vi "Result.vi"(8 "error in (no error)":errorcluster, 10 "Results":T1={"Name"="", "Description"="", "Status"=enum."Passed", "Result Type"=enum."Test Suite", "Execution Time"=0.0, "Data"={"Expected"=variant, "Actual"=variant, "Delta"=variant}}, 11 "Result Model In":refnum<class "Result Model.lvclass">) -> (0 "error out":errorcluster, 3 "Result Model Out":refnum<class "Result Model.lvclass">)   [LabVIEW 2020, in "Result Model.lvclass"]
uses:
  Result Model.lvclass
  Core/Result/Result.ctl
  Core/Result/Status.ctl
  Core/Result/Type.ctl
  Result Model.lvclass/Result Model.ctl
  <vilib>/Utility/miscctls.llb/LVMapReplaceAction.ctl
  Core/Result/Result.lvlib
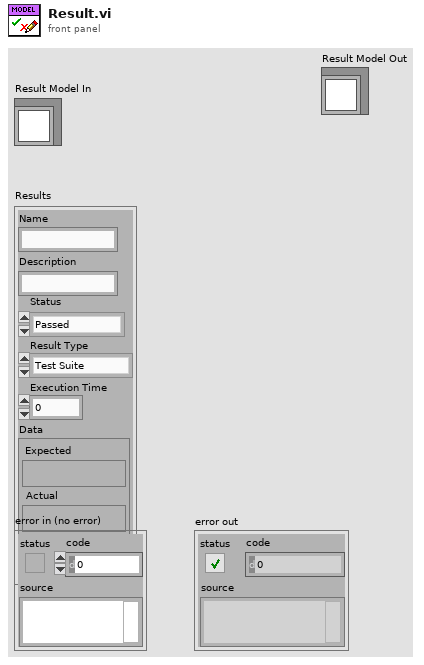
[diagram p1: front panel]
types:
  T1 = typedef "Result.lvlib/Result.ctl" = cluster{"Name":string, "Description":string, "Status":T2, "Result Type":T3, "Execution Time":dbl, "Data":cluster{"Expected":variant, "Actual":variant, "Delta":variant}}
  T2 = typedef "Result.lvlib/Status.ctl" = enum16{"", "Passed", "Failed", "Error", "Skipped", "Setup Error", "Broken", "Teardown Error"}
  T3 = typedef "Result.lvlib/Type.ctl" = enum16{"Test Case", "Test Suite", "Test Run", "Pass", "Fail", "Skip", "Pass if", "Fail if", "Pass if Error", "Fail if Error", "Pass if Equal", "Fail if Equal"}
  T4 = cluster{"Expected":variant, "Actual":variant, "Delta":variant}
  T5 = typedef "LVMapReplaceAction.ctl" = enum32{"Modify Entry only if found", "Add or Modify Entry", "Delete Entry"}
  T6 = cluster{"Result Type":T3, "Status":T2, "Description":string, "Data":cluster{"Expected":variant, "Actual":variant, "Delta":variant}}
  T7 = map{string, cluster{"Result Type":T3, "Status":T2, "Description":string, "Data":cluster{"Expected":variant, "Actual":variant, "Delta":variant}}[]}
  T8 = cluster{"Result Type":T3, "Status":T2, "Description":string, "Data":cluster{"Expected":variant, "Actual":variant, "Delta":variant}}[]
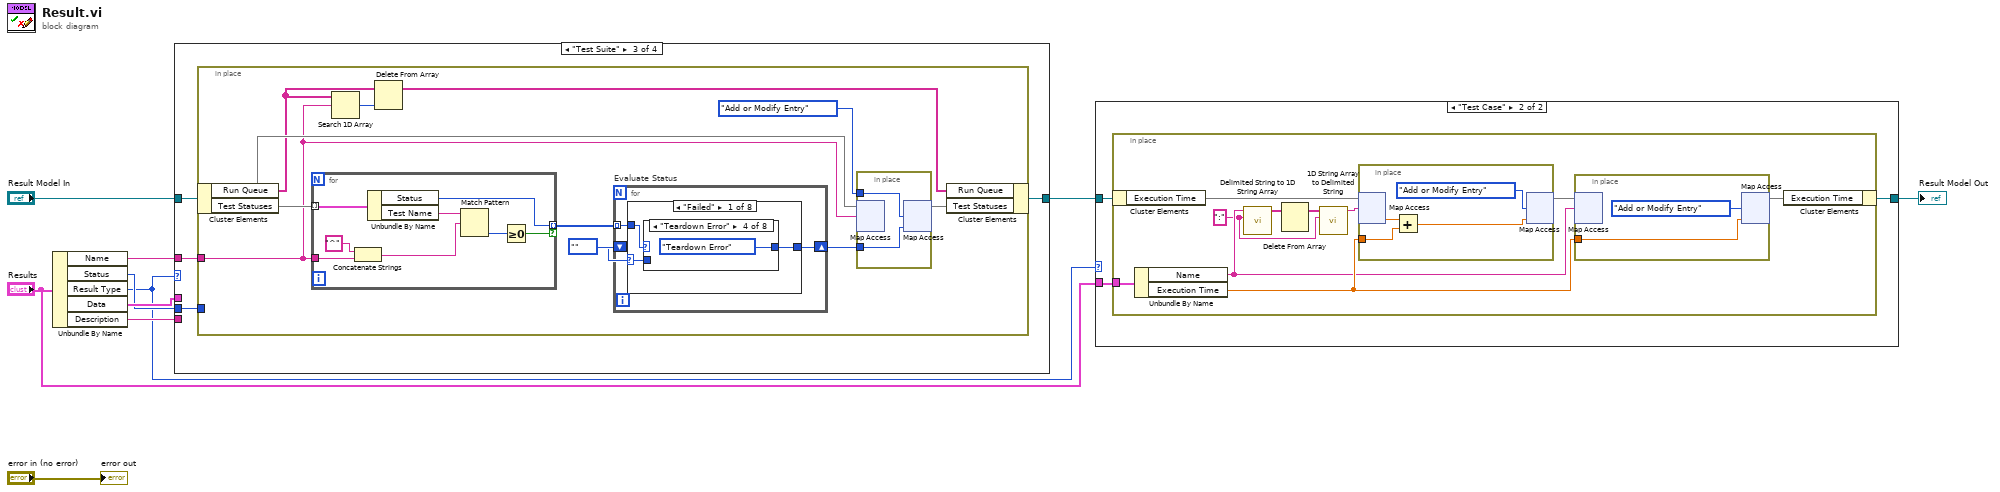
[diagram p0: block diagram]
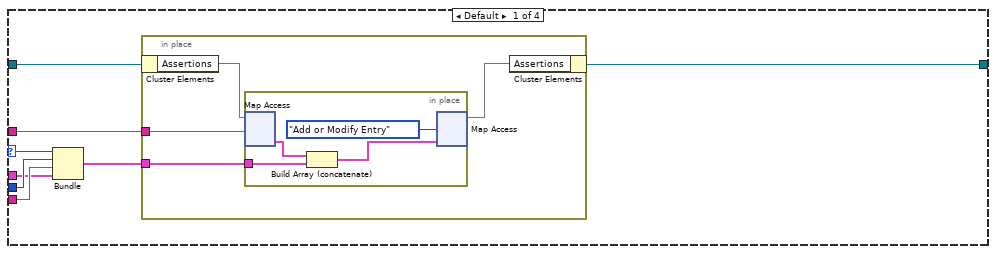
[diagram p2: hidden frame]
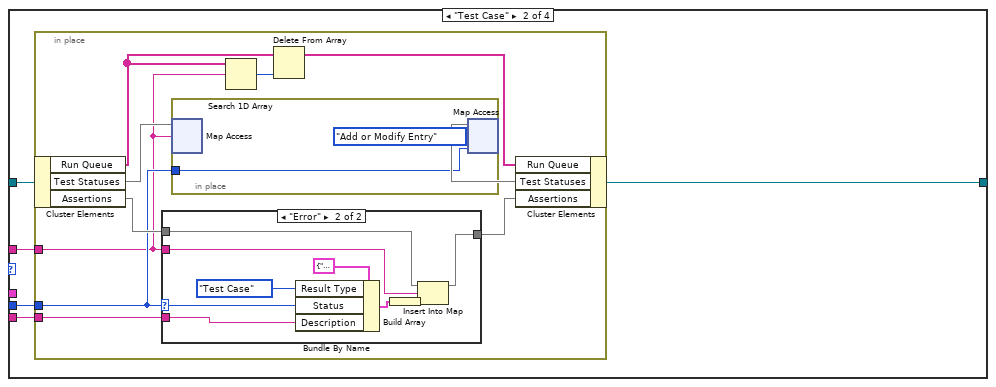
[diagram p3: hidden frame]
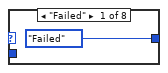
[diagram p5: hidden frame]
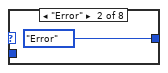
[diagram p6: hidden frame]
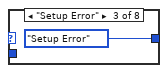
[diagram p7: hidden frame]
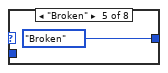
[diagram p8: hidden frame]
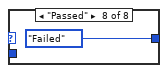
[diagram p11: hidden frame]
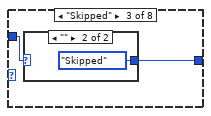
[diagram p13: hidden frame]
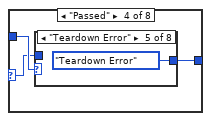
[diagram p15: hidden frame]
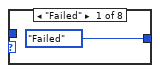
[diagram p16: hidden frame]
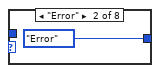
[diagram p17: hidden frame]
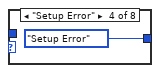
[diagram p19: hidden frame]
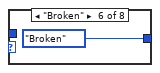
[diagram p20: hidden frame]
diagram:
  n1 = Unbundle By Name("Results") -> ("Name"=w2:string, "Status"=w3:T2, "Result Type"=w1:T3, "Data"=w5:T4, "Description"=w4:string)
  n2 = case shown="\"Test Suite\"" w1 {
    selector: w1 -> [w15 _ _ _]
    tunnel: w2 -> [w16 w31 w57 _]
    tunnel: w3 -> [w14 w30 w56 _]
    tunnel: w4 -> [w17 w27 _ _]
    tunnel: "Result Model In" -> [w13 w29 w55 w126]
    tunnel: [w12 w28 w54 w126] -> w7
    tunnel: w5 -> [w11 _ _ _]
    frame Default {
      n3 = Bundle("Result Type"=w15, "Status"=w14, "Description"=w17, "Data"=w11) -> (w18:T6)  [unwired: 1 in]
      n4 = in-place {
        in-place-border: w18 -> [w22]
        in-place-border: w16 -> [w21]
        n5 = in-place-cluster #1(w13) -> ("Assertions"=w20:T7)
        n6 = in-place {
          in-place-border: w22 -> [w23]
          n7 = in-place-map #2(w20, w21) -> (w26:T8)  [unwired: 1 in, 1 out]
          n8 = Build Array (concatenate)(w26, w23) -> (w25:T8)
          n9 = in-place-map #2(w25, LVMapReplaceAction."Add or Modify Entry" ("action")) -> (w19:T7)  [unwired: 2 out]
        }
        n10 = in-place-cluster #1("Assertions"=w19) -> (w12:refnum<class "Result Model.lvclass">)
      }
    }
    frame "Test Case" {
      n11 = in-place {
        in-place-border: w31 -> [w34]
        in-place-border: w30 -> [w37]
        in-place-border: w27 -> [w36]
        n12 = in-place-cluster #3(w29) -> ("Run Queue"=w33:string[], "Test Statuses"=w41:map{string, T2}, "Assertions"=w39:T7)
        n13 = case shown="\"Error\"" w37 {
          selector: w37 -> [_ w47]
          tunnel: w39 -> [w42 w51]
          tunnel: [w42 w50] -> w38
          tunnel: w34 -> [_ w49]
          tunnel: w36 -> [_ w46]
          frame "", Default {
          }
          frame "Error" {
            n14 = Bundle By Name(cluster=T6 {"Result Type"=enum."Test Case", "Status"=enum."", "Description"="", "Data"={"Expected"=variant, "Actual"=variant, "Delta"=variant}} ("value"), "Result Type"=Type."Test Case", "Status"=w47, "Description"=w46) -> (w44:T6)
            n15 = Build Array(w44) -> (w43:T8)
            n16 = Insert Into Map(map in=w51, key=w49, value=w43) -> (map out=w50:T7)  [unwired: 2 out]
          }
        }
        n17 = in-place {
          in-place-border: w37 -> [w52]
          n18 = in-place-map #4(w41, w34) -> ()  [unwired: 1 in, 2 out]
          n19 = in-place-map #4(w52, LVMapReplaceAction."Add or Modify Entry" ("action")) -> (w40:map{string, T2})  [unwired: 2 out]
        }
        n20 = Search 1D Array(1D array=w33, element=w34) -> (index of element=w35:i32)  [unwired: 1 in]
        n21 = Delete From Array(array=w33, index=w35) -> (array with subset deleted=w32:string[])  [unwired: 1 in, 1 out]
        n22 = in-place-cluster #3("Run Queue"=w32, "Test Statuses"=w40, "Assertions"=w38) -> (w28:refnum<class "Result Model.lvclass">)
      }
    }
    frame "Test Suite" {
      n23 = in-place {
        in-place-border: w57 -> [w58]
        in-place-border: w56 -> [_]
        n24 = in-place-cluster #5(w55) -> ("Run Queue"=w61:string[], "Test Statuses"=w66:map{string, T2})
        n25 = for {
          tunnel: w66 -> [w75] mode=indexing
          tunnel: w58 -> [w73]
          tunnel: [w71] -> w64 mode=indexing if=w70
          n26 = Concatenate Strings("^" ("string"), w73) -> (w69:string)
          n27 = Unbundle By Name(w75) -> ("Status"=w71:T2, "Test Name"=w74:string)
          n28 = Match Pattern(string=w74, regular expression=w69) -> (offset past match=w72:i32)  [unwired: 1 in, 3 out]
          n29 = Greater Or Equal To 0?(x=w72) -> (x >= 0?=w70:bool)
        }
        n30 = Search 1D Array(1D array=w61, element=w58) -> (index of element=w60:i32)  [unwired: 1 in]
        n31 = Delete From Array(array=w61, index=w60) -> (array with subset deleted=w59:string[])  [unwired: 1 in, 1 out]
        n32 = for "Evaluate Status" {
          tunnel: w64 -> [w76] mode=indexing
          shift-right: [w77] -> w63
          shift-left: Status."" ("Current") -> [w78]
          n33 = case shown="\"Failed\"" w78 {
            selector: w78 -> [w79 _ _ w95 w106 _ _ _]
            tunnel: w76 -> [w81 w90 w91 w97 w107 w112 w116 w120]
            tunnel: [w80 w90 w92 w96 w108 w113 w117 w121] -> w77
            frame "Failed" {
              n34 = case shown="\"Teardown Error\"" w81 {
                tunnel: [Status."Failed" ("Merged Status") Status."Error" ("Merged Status") Status."Setup Error" ("Merged Status") Status."Teardown Error" ("Merged Status") Status."Broken" ("Merged Status") w87 w88 Status."Failed" ("Merged Status")] -> w80
                tunnel: w79 -> [_ _ _ _ _ w87 w88 _]
                frame "Failed" {
                }
                frame "Error" {
                }
                frame "Setup Error" {
                }
                frame "Teardown Error" {
                }
                frame "Broken" {
                }
                frame "" {
                }
                frame "Skipped" {
                }
                frame "Passed" {
                }
              }
            }
            frame "" {
            }
            frame "Skipped" {
              n35 = case shown="\"\"" w91 {
                selector: w91 -> [w93 _]
                tunnel: [w93 Status."Skipped" ("Merged Status")] -> w92
                frame Default {
                }
                frame "" {
                }
              }
            }
            frame "Passed" {
              n36 = case shown="\"Teardown Error\"" w97 {
                tunnel: [Status."Failed" ("Merged Status") Status."Error" ("Merged Status") w100 Status."Setup Error" ("Merged Status") Status."Teardown Error" ("Merged Status") Status."Broken" ("Merged Status") Status."Skipped" ("Merged Status") Status."Passed" ("Merged Status")] -> w96
                tunnel: w95 -> [_ _ w100 _ _ _ _ _]
                frame "Failed" {
                }
                frame "Error" {
                }
                frame "" {
                }
                frame "Setup Error" {
                }
                frame "Teardown Error" {
                }
                frame "Broken" {
                }
                frame "Skipped" {
                }
                frame "Passed" {
                }
              }
            }
            frame "Error" {
              n37 = case shown="\"Skipped\"" w107 {
                tunnel: [Status."Skipped" ("Merged Status") w110 Status."Error" ("Merged Status")] -> w108
                tunnel: w106 -> [_ w110 _]
                frame "Skipped" {
                }
                frame "" {
                }
                frame Default {
                }
              }
            }
            frame "Setup Error" {
              n38 = case shown="Default" w112 {
                tunnel: [Status."Skipped" ("Merged Status") Status."Setup Error" ("Merged Status")] -> w113
                frame "Skipped" {
                }
                frame Default {
                }
              }
            }
            frame "Broken" {
              n39 = case shown="\"Setup Error\"" w116 {
                tunnel: [Status."Broken" ("Merged Status") Status."Setup Error" ("Merged Status")] -> w117
                frame Default {
                }
                frame "Setup Error" {
                }
              }
            }
            frame "Teardown Error" {
              n40 = case shown="\"Skipped\"" w120 {
                tunnel: [Status."Skipped" ("Merged Status") Status."Teardown Error" ("Merged Status")] -> w121
                frame "Skipped" {
                }
                frame Default {
                }
              }
            }
          }
        }
        n41 = in-place {
          in-place-border: LVMapReplaceAction."Add or Modify Entry" ("action") -> [w125]
          in-place-border: w63 -> [w124]
          n42 = in-place-map #6(w66, w58) -> ()  [unwired: 1 in, 2 out]
          n43 = in-place-map #6(w124, w125) -> (w67:map{string, T2})  [unwired: 2 out]
        }
        n44 = in-place-cluster #5("Run Queue"=w59, "Test Statuses"=w67) -> (w54:refnum<class "Result Model.lvclass">)
      }
    }
    frame "Test Run" {
    }
  }
  n45 = case shown="\"Test Case\"" w1 {
    tunnel: "Results" -> [_ w130]
    tunnel: w7 -> [w127 w128]
    tunnel: [w127 w129] -> w6
    frame Default {
    }
    frame "Test Case" {
      n46 = in-place {
        in-place-border: w130 -> [w139]
        w131 = ":" ("delimiter")
        n47 = in-place-cluster #7(w128) -> ("Execution Time"=w135:map{string, dbl})
        n48 = Unbundle By Name(w139) -> ("Name"=w137:string, "Execution Time"=w138:dbl)
        n49 = call <vilib>:"Delimited String to 1D String Array.vi"("delimiter"=w131, "delimited string"=w137) -> ("string array"=w133:string[])  [unwired: 9 in]
        n50 = Delete From Array(array=w133) -> (array with subset deleted=w132:string[])  [unwired: 2 in, 1 out]
        n51 = call <vilib>:"1D String Array to Delimited String.vi"("delimiter"=w131, "string array"=w132) -> ("delimited string"=w136:string)  [unwired: 9 in]
        n52 = in-place {
          in-place-border: w138 -> [w144]
          n53 = in-place-map #8(w135, w136) -> (w143:dbl)  [unwired: 1 in, 1 out]
          n54 = Add(x=w143, y=w144) -> (x+y=w146:dbl)
          n55 = in-place-map #8(w146, LVMapReplaceAction."Add or Modify Entry" ("action")) -> (w140:map{string, dbl})  [unwired: 2 out]
        }
        n56 = in-place {
          in-place-border: w138 -> [w141]
          n57 = in-place-map #9(w140, w137) -> ()  [unwired: 1 in, 2 out]
          n58 = in-place-map #9(w141, LVMapReplaceAction."Add or Modify Entry" ("action")) -> (w134:map{string, dbl})  [unwired: 2 out]
        }
        n59 = in-place-cluster #7("Execution Time"=w134) -> (w129:refnum<class "Result Model.lvclass">)
      }
    }
  }
  "Result Model Out" <- w6
  "error out" <- "error in (no error)"
